vi "el_instrumento_virtual_con_otro_nombre_eta_funciona.vi"() -> ()   [LabVIEW 2009]
uses:
  <vilib>/Analysis/3filter.llb/Butterworth Filter (DBL).vi
  <vilib>/Analysis/NI_AALBase.lvlib
  <vilib>/Analysis/NI_AALPro.lvlib
panel:
  out "count":i32
  out "BPM":dbl
  out "Señal filtrada corregida":cluster{"Y":dbl[], "Y":dbl[]}[](graph)
  in  "low cutoff freq: fh 3":ext=0.45000000000000007 format="%0.6f"
  out "Línea basal":cluster{"Y":dbl[], "Y":dbl[]}[](graph)
  in  "high cutoff freq: fh 3":ext=0.45000000000000007 format="%0.6f"
  in  "low cutoff freq: fh 2":ext=0.45000000000000007 format="%0.6f"
  out "Señal filtrada":cluster{"Y":dbl[], "Y":dbl[]}[](graph)
  out "Señal sin filtrar":cluster{"Y":dbl[], "Y":dbl[]}[](graph)
  in  "Begin Sample 2":i32 caption="Begin Sample"
  in  "Number of Samples 2":dbl=6000.0
  in  "Scan Rate (Hz) 2":dbl=1000.0
  in  "Range Constants 2":u8[](array[ring])=[1, 1] items=["LJ_rgBIP10V", "LJ_rgBIP1V", "LJ_rgBIPP1V", "LJ_rgBIPP01V"]
  # "Escoger los dos primeros\nelementos de la lista\npara ajustar el margen\ndinámico (de arriba a abajo,\n 10 V, 1 V, 0,1 V y 0,01 V)."
  # "EJEMPLO CON UN FILTRO PASO BAJO"
  # "Señal filtrada"
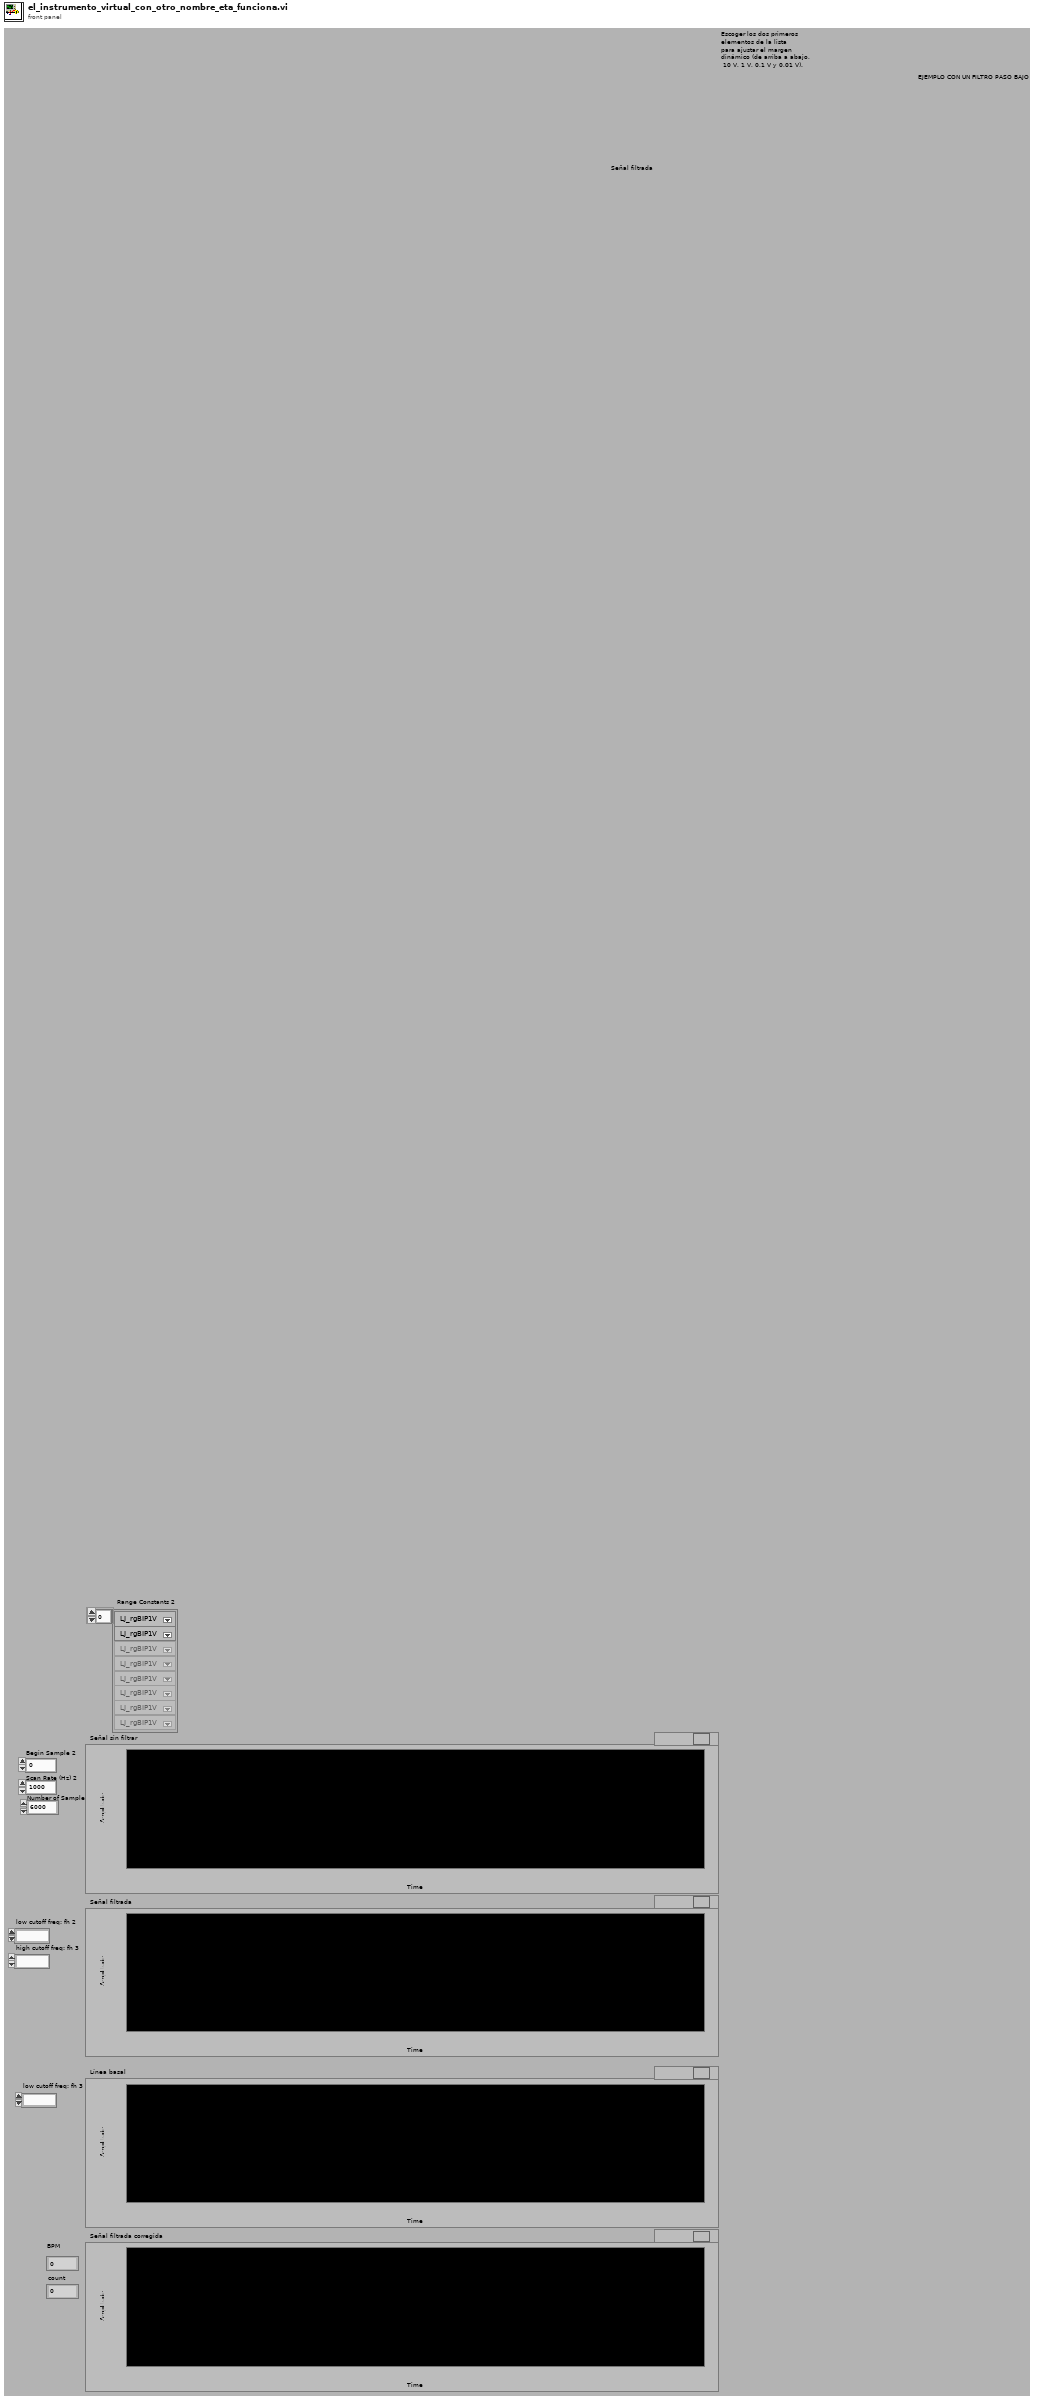
[diagram p1: front panel]
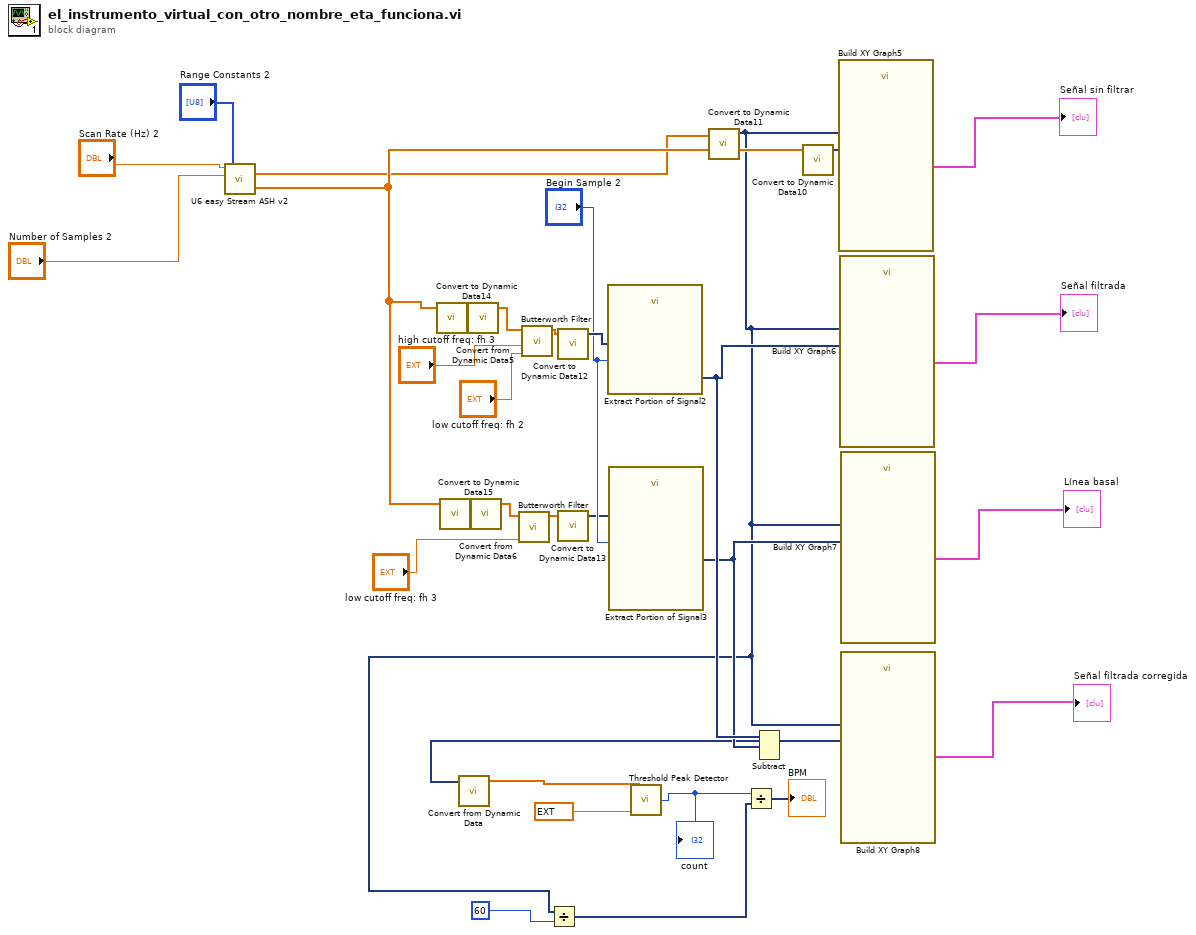
[diagram p0: block diagram]
diagram:
  n1 = call "U6 easy Stream ASH v2.vi"("Range Constants"="Range Constants 2", "Number of Samples"="Number of Samples 2", "Scan Rate (Hz)"="Scan Rate (Hz) 2") -> ("Tiempo"=w9:dbl[], "Señal"=w15:dbl[])  [unwired: 3 in]
  n2 = call "Convert to Dynamic Data14"("Array"=w15) -> ("Dynamic Data Type"=w23:dynamicdata)  [unwired: 3 in]
  n3 = call "Convert to Dynamic Data15"("Array"=w15) -> ("Dynamic Data Type"=w22:dynamicdata)  [unwired: 3 in]
  n4 = call "Convert from Dynamic Data5"("Dynamic Data Type"=w23) -> ("Array"=w27:dbl[])  [unwired: 3 in]
  n5 = call "Convert from Dynamic Data6"("Dynamic Data Type"=w22) -> ("Array"=w25:dbl[])  [unwired: 3 in]
  n6 = call-poly <vilib>:"Butterworth Filter.vi"("low cutoff freq: fl"="low cutoff freq: fh 3", "X"=w25) -> ("Filtered X"=w19:dbl[])  [unwired: 6 in, 1 out]
  n7 = call-poly <vilib>:"Butterworth Filter.vi"("low cutoff freq: fl"="low cutoff freq: fh 2", "high cutoff freq: fh"="high cutoff freq: fh 3", "X"=w27) -> ("Filtered X"=w21:dbl[])  [unwired: 5 in, 1 out]
  n8 = call "Convert to Dynamic Data12"("Array"=w21) -> ("Dynamic Data Type"=w20:dynamicdata)  [unwired: 3 in]
  n9 = call "Convert to Dynamic Data13"("Array"=w19) -> ("Dynamic Data Type"=w12:dynamicdata)  [unwired: 3 in]
  n10 = call "Extract Portion of Signal2"("Begin Sample"="Begin Sample 2", "Signals"=w20) -> ("Section"=w16:dynamicdata)  [unwired: 8 in, 1 out]
  n11 = call "Extract Portion of Signal3"("Begin Sample"="Begin Sample 2", "Signals"=w12) -> ("Section"=w14:dynamicdata)  [unwired: 8 in, 1 out]
  n12 = call "Convert to Dynamic Data11"("Array"=w9) -> ("Dynamic Data Type"=w3:dynamicdata)  [unwired: 3 in]
  n13 = Divide(x=w3, y=60) -> (x/y=w1:dynamicdata)
  n14 = Subtract(1:w14, 2:w16) -> (0:w11:dynamicdata)  [unwired: 1 in, 1 out]
  n15 = call "Convert from Dynamic Data"("Dynamic Data Type"=w11) -> ("Array"=w7:dbl[])  [unwired: 3 in]
  n16 = call <vilib>:"Threshold Peak Detector.vi"("threshold"=ext 0.03 ("width"), "X"=w7) -> ("count"=w2:i32)  [unwired: 1 in, 2 out]
  "count" <- w2
  n17 = Divide(x=w2, y=w1) -> (x/y=→"BPM":dynamicdata)
  n18 = call "Convert to Dynamic Data10"("Array"=w15) -> ("Dynamic Data Type"=w24:dynamicdata)  [unwired: 3 in]
  n19 = call "Build XY Graph5"("Y Input"=w24, "X Input"=w3) -> ("XY Graph"=→"Señal sin filtrar":cluster{"Y":dbl[], "Y":dbl[]}[])  [unwired: 8 in, 1 out]
  n20 = call "Build XY Graph6"("Y Input"=w16, "X Input"=w3) -> ("XY Graph"=→"Señal filtrada":cluster{"Y":dbl[], "Y":dbl[]}[])  [unwired: 8 in, 1 out]
  n21 = call "Build XY Graph7"("Y Input"=w14, "X Input"=w3) -> ("XY Graph"=→"Línea basal":cluster{"Y":dbl[], "Y":dbl[]}[])  [unwired: 8 in, 1 out]
  n22 = call "Build XY Graph8"("Y Input"=w11, "X Input"=w3) -> ("XY Graph"=→"Señal filtrada corregida":cluster{"Y":dbl[], "Y":dbl[]}[])  [unwired: 8 in, 1 out]
